vi "CAENHV Get Exec Comm List.vi"(8 "error in (no error)":errorcluster, 11 "handle":i32) -> (0 "error out":errorcluster, 2 "CommNameList":string[](array[string]), 3 "NumComm":u16)   [LabVIEW 2018, in "CAENHVWrapper.lvlib"]
doc: "CAENHVLIB_API CAENHVRESULT CAENHV_GetExecCommList(int handle,\n ushort *NumComm, char **CommNameList);"
uses:
  <instrlib>/CAENHVWrapper/CAENHVWrapper.lvlib
  <vilib>/Utility/importsl/GetValueByPointer/datatype.ctl
  <vilib>/Utility/importsl/GetValueByPointer/GetValueByPointer.xnode
  <instrlib>/CAENHVWrapper/VIs/CAENHVWrapper.dll
  <resource>/lvimptsl.dll
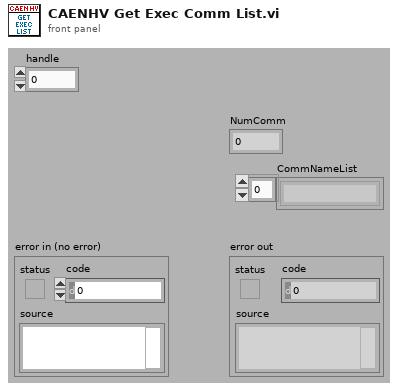
[diagram p1: front panel]
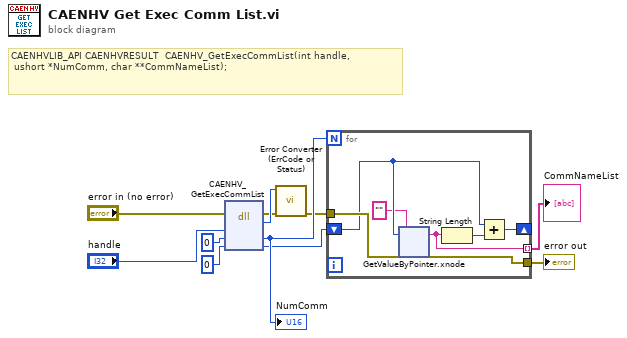
[diagram p0: block diagram]
diagram:
  # "CAENHVLIB_API CAENHVRESULT  CAENHV_GetExecCommList(int handle,\n ushort *NumComm, char **CommNameList);"
  n1 = dll-call lib="C:/Program Files (x86)/National Instruments/LabVIEW 2018/instr.lib/CAENHVWrapper/VIs/CAENHVWrapper.*" fn="CAENHV_GetExecCommList"(error in="error in (no error)", "handle"="handle", "NumComm"=u16 0, "CommNameList"=i64 0) -> (error out=w8:errorcluster, "return type"=w9:i32, "NumComm"=w6:u16, "CommNameList"=w5:i64)  [unwired: 3 in, 1 out]
  "NumComm" <- w6
  n2 = call <instrlib>:"Error Converter (ErrCode or Status).vi"("error in (no error)"=w8, "error code"=w9) -> ("error out"=w4:errorcluster)  [unwired: 9 in]
  n3 = for {
    N: w6 -> [_]
    shift-right: [w14] -> _
    shift-left: w5 -> [w16]
    tunnel: w4 -> [w18]
    tunnel: [w17] -> w3
    tunnel: [w12] -> w2 mode=indexing
    n4 = xnode "GetValueByPointer.xnode"("Pointer"=w16, "InputType"="", "ErrorIn"=w18) -> ("Output"=w12:string, "ErrorOut"=w17:errorcluster)  [unwired: 1 in]
    n5 = String Length(string=w12) -> (length=w15:i32)
    n6 = Add(x=w16, y=w15) -> (x+y=w14:i64)
  }
  "error out" <- w3
  "CommNameList" <- w2
